vi "chartsheet set chart.vi"(8 "error in (no error)":errorcluster, 10 "chart":u32, 11 "chartsheet":u32) -> (0 "error out":errorcluster, 3 "function return":u32(ring))   [LabVIEW 8.6]
doc: "lxw_error chartsheet_set_chart(lxw_chartsheet chartsheet, lxw_chart chart);"
uses:
  pending_lvxlsxwriter/xlsxwriter.dll
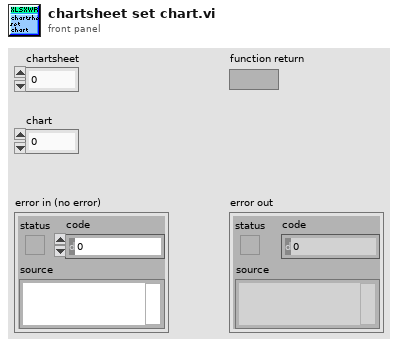
[diagram p1: front panel]
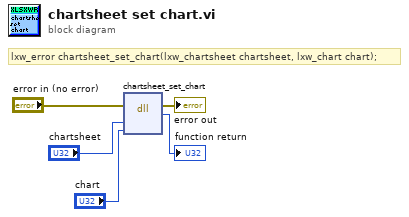
[diagram p0: block diagram]
diagram:
  # "lxw_error chartsheet_set_chart(lxw_chartsheet chartsheet, lxw_chart chart);"
  n1 = dll-call lib="C:/Users/WDAGUtilityAccount/Desktop/pending_lvxlsxwriter/xlsxwriter.*" fn="chartsheet_set_chart"(error in="error in (no error)", "chartsheet"="chartsheet", "chart"="chart") -> (error out=→"error out":errorcluster, →"function return":u32)  [unwired: 4 in, 1 out]
